vi "PXI-Pause-Kill Counter.vi"(0 "Counter Task":T1, 7 "Pause":bool, 11 "error in (no error)":errorcluster) -> (15 "error out":errorcluster)   [LabVIEW 2015]
uses:
  Type Defs/Task Struct.ctl
  PXI Globals.vi
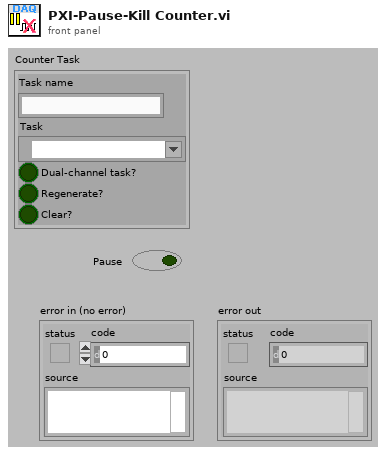
[diagram p1: front panel]
types:
  T1 = typedef "Task Struct.ctl" = cluster{"Task name":string, "Task":refnum<k21>, "Dual-channel task?":bool, "Regenerate?":bool, "Clear?":bool}
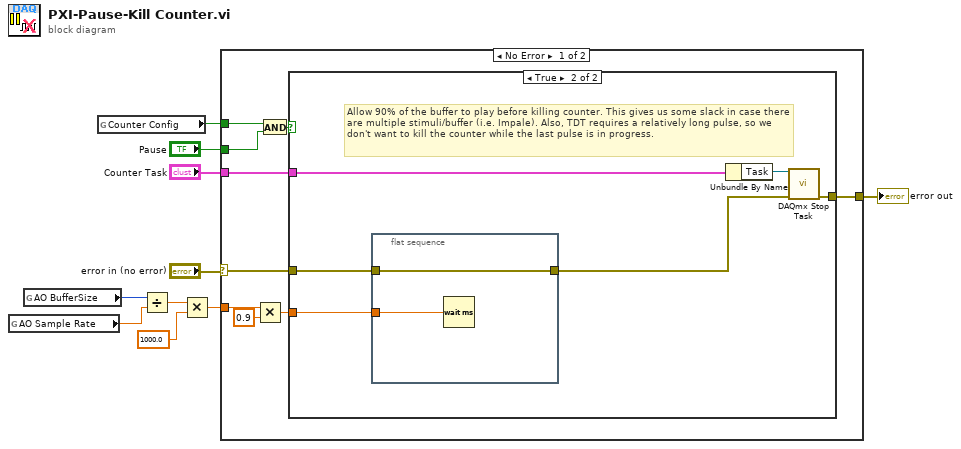
[diagram p0: block diagram]
diagram:
  n1 = global read "PXI Globals.vi" "AO Sample Rate"() -> (w3:dbl)
  n2 = global read "PXI Globals.vi" "AO BufferSize"() -> (w5:i32)
  n3 = global read "PXI Globals.vi" "Counter Config"() -> (w7:bool)
  n4 = Divide(x=w5, y=w3) -> (x/y=w4:dbl)
  n5 = Multiply(x=w4, y=1000.0) -> (x*y=w2:dbl)
  n6 = case shown="No Error" "error in (no error)" {
    selector: "error in (no error)" -> [w19 w29]
    tunnel: [w18 w29] -> w9
    tunnel: "Counter Task" -> [w17 _]
    tunnel: w7 -> [w15 _]
    tunnel: "Pause" -> [w14 _]
    tunnel: w2 -> [w13 _]
    frame No Error {
      n7 = Multiply(x=w13, y=0.9) -> (x*y=w11:dbl)
      n8 = And(x=w15, y=w14) -> (x .and. y?=w16:bool)
      n9 = case shown="True" w16 {
        tunnel: w19 -> [w20 w22]
        tunnel: [w20 w26] -> w18
        tunnel: w17 -> [_ w25]
        tunnel: w11 -> [_ w23]
        frame False {
        }
        frame True {
          # "Allow 90% of the buffer to play before killing counter. This gives us some slack in case there are multiple stimuli/buffer (i.e. Impale). Also, TDT requires a relatively long pulse, so we don't want to kill the counter while the last pulse is in progress."
          n10 = flat-sequence {
            tunnel: w23 -> [w28]
            tunnel: w22 -> [w27]
            tunnel: [w27] -> w21
            frame #0 {
              n11 = Wait (ms)(milliseconds to wait=w28) -> ()  [unwired: 1 out]
            }
          }
          n12 = Unbundle By Name(w25) -> ("Task"=w24:refnum<k21>)
          n13 = call <vilib>:"DAQmx Stop Task.vi"("task/channels in"=w24, "error in"=w21) -> ("error out"=w26:errorcluster)  [unwired: 12 in, 1 out]
        }
      }
    }
    frame Error {
    }
  }
  "error out" <- w9
